vi "Append VI Block Diagram to Report (refnum).vi"(0 "report in":refnum<class "NI_report.lvclass">, 1 "hidden frames":bool, 2 "image format (jpeg)":enum32{"PNG", "JPEG", "GIF"}(ring)=enum."JPEG", 5 "VI":refnum<vi>, 9 "alignment (default)":T2, 11 "error in (no error)":errorcluster, 12 "ordered (repeat from higher level if nested)":bool, 13 "MS Office parameters":T1) -> (4 "report out":refnum<class "NI_report.lvclass">, 6 "VI out":refnum<vi>, 8 "start out (Word)":i32, 10 "end out (Word)":i32, 15 "error out":errorcluster)   [LabVIEW 2020, in "NI_ReportGenerationCore.lvlib"]
doc: "Creates an image of the block diagram of the VI you specify in <B>VI</B> and appends the image to a report. Wire data to the <B>VI</B> input to determine the polymorphic instance to use or manually select the instance."
uses:
  <vilib>/Utility/NIReport.llb/NI_ReportGenerationCore.lvlib
  <vilib>/Utility/NIReport.llb/NI_report.lvclass
  <vilib>/Utility/NIReport.llb/HTML Report Image Alignment.ctl
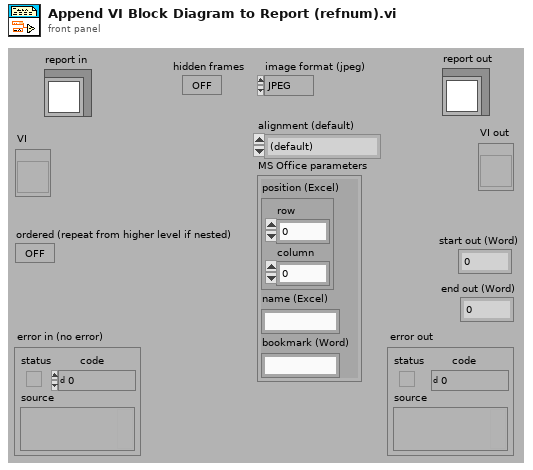
[diagram p1: front panel]
types:
  T1 = cluster{"position (Excel)":cluster{"row":i32, "column":i32}, "name (Excel)":string, "bookmark (Word)":string}
  T2 = typedef "NI_ReportGenerationCore.lvlib/HTML Report Image Alignment.ctl" = enum16{"(default)", "LEFT", "RIGHT", "TOP", "TEXTTOP", "MIDDLE", "ABSMIDDLE", "BASELINE", "BOTTOM", "ABSBOTTOM"}
  T3 = enum32{"invalid app kind", "Development System", "Run Time System", "Student Edition", "Embedded LabVIEW", "Evaluation", "Custom"}
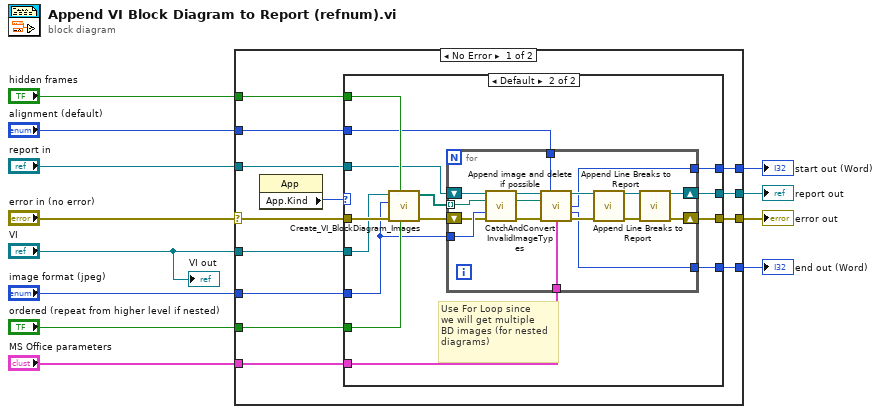
[diagram p0: block diagram]
diagram:
  n1 = case shown="No Error" "error in (no error)" {
    selector: "error in (no error)" -> [w25 w60]
    tunnel: [w21 w60] -> w11
    tunnel: [w14 w59] -> w9
    tunnel: "report in" -> [w15 w59]
    tunnel: "VI" -> [w24 _]
    tunnel: "image format (jpeg)" -> [w16 _]
    tunnel: "hidden frames" -> [w23 _]
    tunnel: "ordered (repeat from higher level if nested)" -> [w22 _]
    tunnel: "alignment (default)" -> [w20 _]
    tunnel: "MS Office parameters" -> [w19 _]
    tunnel: [w18 _] -> w2
    tunnel: [w17 _] -> w1
    frame No Error {
      n2 = property class="App"() -> ("App.Kind"=w13:T3)  [unwired: 2 in, 2 out]
      n3 = case shown="Default" w13 {
        tunnel: w25 -> [w27 w41]
        tunnel: w24 -> [_ w40]
        tunnel: w23 -> [_ w37]
        tunnel: w22 -> [_ w36]
        tunnel: [w27 w35] -> w21
        tunnel: w20 -> [_ w34]
        tunnel: w19 -> [_ w33]
        tunnel: [_ w32] -> w18
        tunnel: [_ w31] -> w17
        tunnel: w16 -> [_ w30]
        tunnel: w15 -> [w26 w29]
        tunnel: [w26 w28] -> w14
        frame "Run Time System" {
          # "Do not try to append\ndiagram if running\nin an executable"
        }
        frame Default {
          # "Use For Loop since\nwe will get multiple\nBD images (for nested\ndiagrams)"
          n4 = call <vilib>:"Create_VI_BlockDiagram_Images.vi"("Printing:Custom Diagram Repeat?"=w36, "Printing:Custom Diagram Hidden?"=w37, "error in (no error)"=w41, "Image Format (jpeg)"=w30, "VI"=w40) -> ("error out"=w38:errorcluster, "Paths to images"=w39:path[])  [unwired: 5 in]
          n5 = for {
            tunnel: w39 -> [w53] mode=indexing
            shift-right: [w54] -> w35
            shift-left: w38 -> [w51]
            tunnel: w30 -> [w52]
            tunnel: w34 -> [w48]
            tunnel: w33 -> [w47]
            tunnel: [w46] -> w32
            tunnel: [w45] -> w31
            shift-right: [w42] -> w28
            shift-left: w29 -> [w44]
            n6 = call-dynamic "CatchAndConvertInvalidImageTypes.vi"("report in"=w44, "path to image"=w53, "image format (jpeg)"=w52, "error in (no error)"=w51) -> ("report out"=w43:refnum<class "NI_report.lvclass">, "path to image out"=w49:path, "error out"=w50:errorcluster)  [unwired: 9 in]
            n7 = call-dynamic "Append image and delete if possible.vi"("report in"=w43, "alignment (default)"=w48, "path to image"=w49, "error in (no error)"=w50, "MS Office parameters"=w47) -> ("report out"=w57:refnum<class "NI_report.lvclass">, "start out Word)"=w46:i32, "end out Word)"=w45:i32, "error out"=w58:errorcluster)  [unwired: 7 in]
            n8 = call <vilib>:"Append Line Breaks to Report.vi"("report in"=w57, "error in (no error)"=w58) -> ("report out"=w55:refnum<class "NI_report.lvclass">, "error out"=w56:errorcluster)  [unwired: 12 in]
            n9 = call <vilib>:"Append Line Breaks to Report.vi"("report in"=w55, "error in (no error)"=w56) -> ("report out"=w42:refnum<class "NI_report.lvclass">, "error out"=w54:errorcluster)  [unwired: 12 in]
          }
        }
      }
    }
    frame Error {
    }
  }
  "error out" <- w11
  "report out" <- w9
  "start out (Word)" <- w2
  "end out (Word)" <- w1
  "VI out" <- "VI"
